vi "Init.vi"(8 "error in (no error)":errorcluster, 11 "PowerSupply in":refnum<class "PowerSupply.lvclass">) -> (0 "error out":errorcluster, 3 "PowerSupply out":refnum<class "PowerSupply.lvclass">)   [LabVIEW 2020, in "LAF2024Q2.lvlib" / "PowerSupply.lvclass"]
uses:
  PowerSupply.lvclass
  PowerSupply.lvclass/PowerSupply.ctl
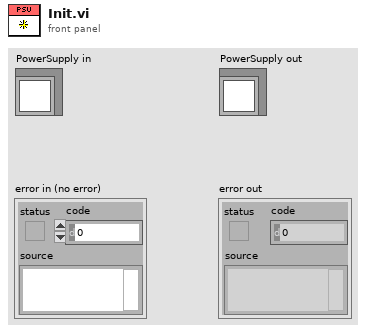
[diagram p1: front panel]
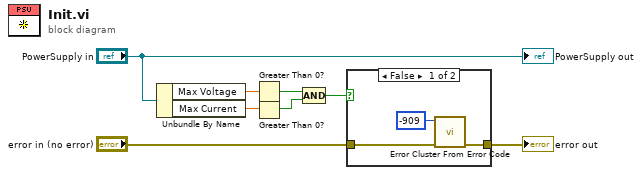
[diagram p0: block diagram]
diagram:
  n1 = Unbundle By Name("PowerSupply in") -> ("Max Voltage"=w7:dbl, "Max Current"=w6:dbl)
  n2 = Greater Than 0?(x=w7) -> (x > 0?=w5:bool)
  n3 = Greater Than 0?(x=w6) -> (x > 0?=w4:bool)
  n4 = Compound Arithmetic op=AND(w5, w4) -> (w2:bool)
  n5 = case shown="False" w2 {
    tunnel: "error in (no error)" -> [w11 w12]
    tunnel: [w10 w12] -> w1
    frame False {
      n6 = call <vilib>:"Error Cluster From Error Code.vi"("error in (no error)"=w11, "error code (0)"=-909) -> ("error out"=w10:errorcluster)  [unwired: 7 in]
    }
    frame True {
      # "Good!"
    }
  }
  "error out" <- w1
  "PowerSupply out" <- "PowerSupply in"
